vi "Default Instrument Setup.vi"(8 "error in (no error)":errorcluster, 11 "VISA resource name":refnum<visa-resource-name>) -> (0 "error out":errorcluster, 3 "VISA resource name out":refnum<visa-resource-name>)   [LabVIEW 2019, in "Andeen-Hagerling 2700(400 firmware).lvlib"]
doc: "This Utility VI sends a default command string to the instrument whenever a new VISA session is opened, or the instrument is reset. Use this VI as a subVI for the Initialize and Reset VIs. Altering this VI could cause these two VIs to operate incorrectly.\n\nThis VI configures the bridge for performing programmatic control. This includes turning off serial echo, labels, and setting error messages to numeric code, and turning on the Sample Swtich field."
uses:
  Andeen-Hagerling 2700(400 firmware).lvlib
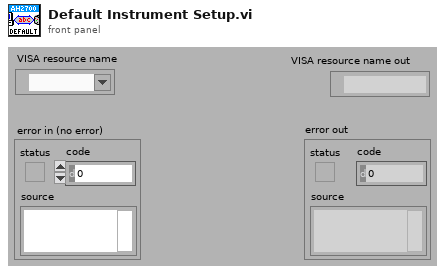
[diagram p1: front panel]
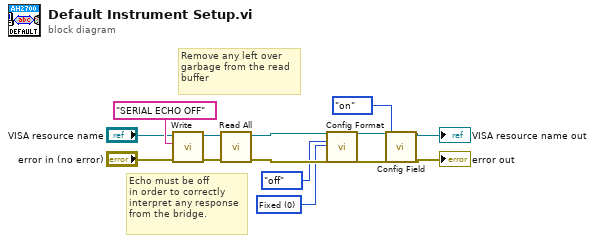
[diagram p0: block diagram]
diagram:
  w6 = u16 0 items=["Fixed", "Variable"] ("Field Width (fixed)")
  # "Echo must be off\nin order to correctly\ninterpret any response\nfrom the bridge."
  # "Remove any left over\ngarbage from the read\nbuffer"
  n1 = call "Write.vi"("error in"="error in (no error)", "command"="SERIAL ECHO OFF", "VISA resource name"="VISA resource name") -> ("error out"=w10:errorcluster, "VISA resource name out"=w11:refnum<visa-resource-name>)  [unwired: 7 in]
  n2 = call "Read All.vi"("error in"=w10, "VISA resource name"=w11) -> ("error out"=w8:errorcluster, "VISA resource name out"=w9:refnum<visa-resource-name>)  [unwired: 7 in, 1 out]
  n3 = call "Config Format.vi"("VISA resource name"=w9, "Lasbelling (on)"=enum16{"off", "on"}."off", "Field Width (fixed)"=w6, "error in"=w8) -> ("VISA resource name out"=w5:refnum<visa-resource-name>, "error out"=w4:errorcluster)  [unwired: 22 in]
  n4 = call "Config Field.vi"("VISA resource name"=w5, "error in"=w4, "Sample (off)"=enum16{"off", "on"}."on") -> ("VISA resource name out"=→"VISA resource name out":refnum<visa-resource-name>, "error out"=→"error out":errorcluster)  [unwired: 23 in]
